vi "BSC To More Generic Example.vi"() -> ()   [LabVIEW 2011]
uses:
  C:/Users/kmuraszko/Documents/Thorlabs/Motor VI/Kinesis LabVIEW/Working KPA101 Code!/Thorlabs.MotionControl.Controls.dll
  Kinesis LabVIEW/Working KPA101 Code!/Thorlabs.MotionControl.Controls.dll
  C:/Users/kmuraszko/Documents/Thorlabs/Motor VI/Kinesis LabVIEW/Working KPA101 Code!/Thorlabs.MotionControl.Benchtop.StepperMotorCLI.dll
  Kinesis LabVIEW/Working KPA101 Code!/Thorlabs.MotionControl.Benchtop.StepperMotorCLI.dll
  C:/Users/kmuraszko/Documents/Thorlabs/Motor VI/Kinesis LabVIEW/Working KPA101 Code!/Thorlabs.MotionControl.GenericMotorCLI.dll
  Kinesis LabVIEW/Working KPA101 Code!/Thorlabs.MotionControl.GenericMotorCLI.dll
panel:
  in  "SerialNumber":string
  in  "stop":bool
  in  "BenchtopStepperControl":refnum<k24>(container)
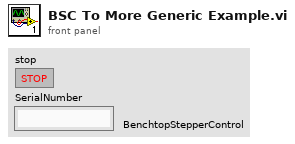
[diagram p1: front panel]
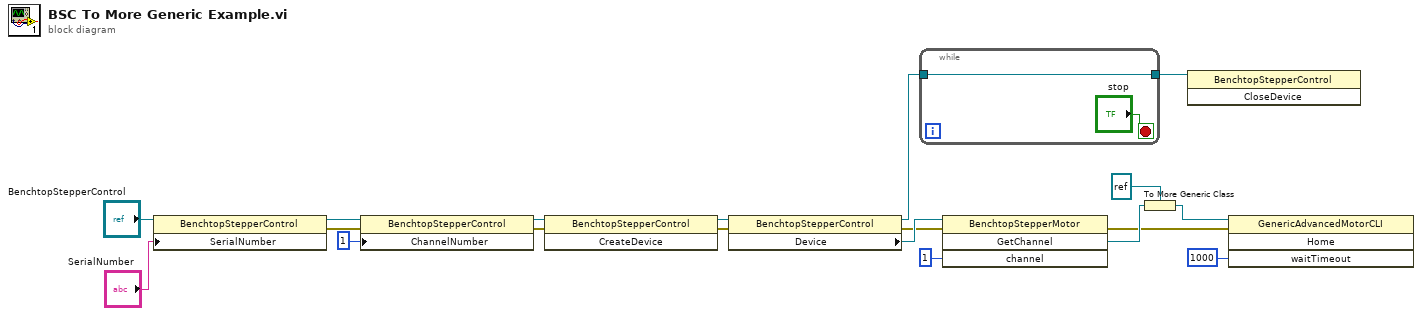
[diagram p0: block diagram]
diagram:
  n1 = property class="BenchtopStepperControl"(reference="BenchtopStepperControl", "SerialNumber"="SerialNumber") -> (reference out=w18:refnum<k24>, error out=w6:errorcluster)  [unwired: 1 in]
  n2 = property class="BenchtopStepperControl"(reference=w18, error in=w6, "ChannelNumber"=1) -> (reference out=w17:refnum<k24>, error out=w5:errorcluster)
  n3 = invoke class="BenchtopStepperControl" method="CreateDevice"(reference=w17, error in=w5) -> (reference out=w15:refnum<k24>, error out=w4:errorcluster)  [unwired: 1 in, 1 out]
  n4 = property class="BenchtopStepperControl"(reference=w15, error in=w4) -> (reference out=w12:refnum<k24>, error out=w3:errorcluster, "Device"=w14:refnum<k24>)
  n5 = while {
    tunnel: [w20] -> w13
    tunnel: w12 -> [w20]
    stop <- "stop" stop-if-true
  }
  n6 = invoke class="BenchtopStepperMotor" method="GetChannel"(reference=w14, error in=w3, "channel"=i16 1) -> (error out=w2:errorcluster, "GetChannel"=w10:refnum<k24>)  [unwired: 1 in, 2 out]
  n7 = To More Generic Class(target class=refnum<k24> refnum, reference=w10) -> (generic class reference=w9:refnum<k24>)
  n8 = invoke class="BenchtopStepperControl" method="CloseDevice"(reference=w13) -> ()  [unwired: 2 in, 3 out]
  n9 = invoke class="GenericAdvancedMotorCLI" method="Home"(reference=w9, error in=w2, "waitTimeout"=1000) -> ()  [unwired: 1 in, 4 out]
